vi "run.vi"(8 "error in (no error)":errorcluster, 10 "Path":path, 11 "ConsoleViewer in":refnum<class "ConsoleViewer.lvclass">) -> (0 "error out":errorcluster, 3 "ConsoleViewer out":refnum<class "ConsoleViewer.lvclass">)   [LabVIEW 2009, in "Views.lvlib" / "ConsoleViewer.lvclass"]
uses:
  ConsoleViewer.lvclass
  Tools/CommandProcessor/CommandProcessor.lvclass
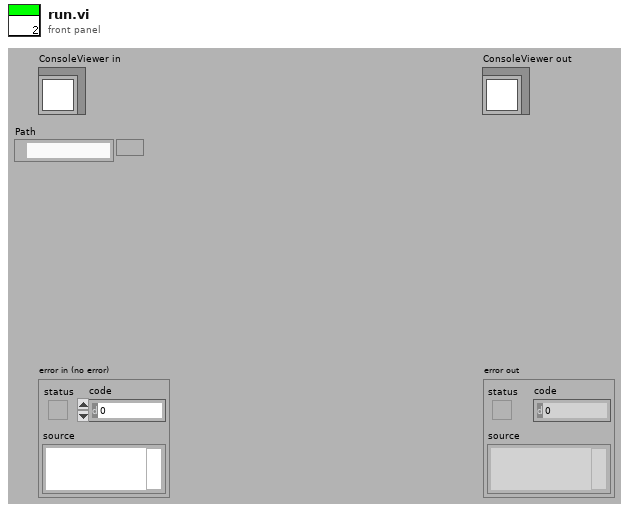
[diagram p1: front panel]
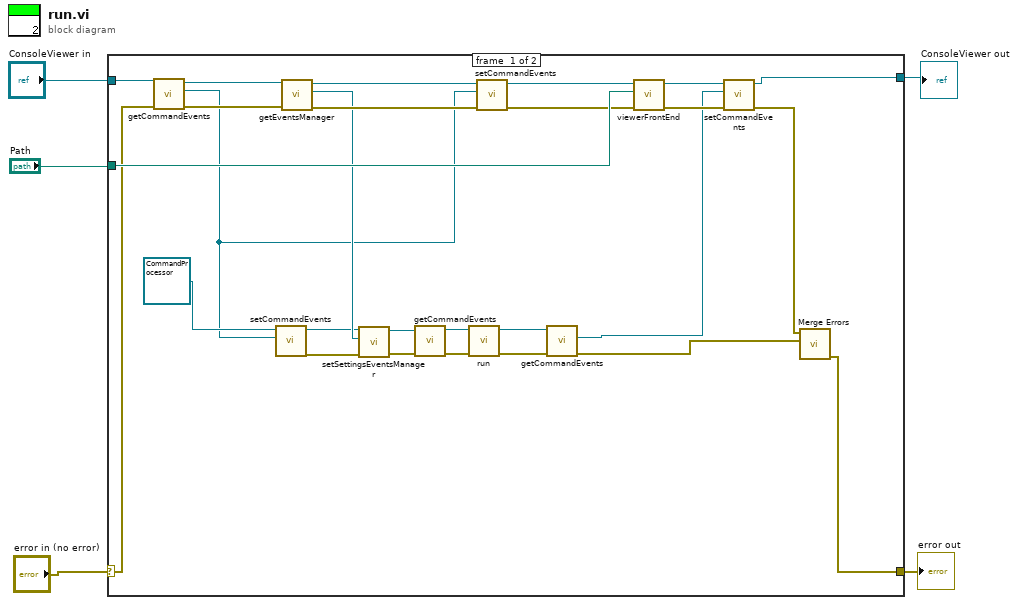
[diagram p0: block diagram]
diagram:
  n1 = case shown="No Error" "error in (no error)" {
    selector: "error in (no error)" -> [w17 w33]
    tunnel: "ConsoleViewer in" -> [w18 w34]
    tunnel: [w9 w34] -> w4
    tunnel: "Path" -> [w32 _]
    tunnel: [w31 w33] -> w1
    frame #0 {
      n2 = call-dynamic "getCommandEvents.vi"("error in (no error)"=w17, "ConsoleViewer.lvclass in"=w18) -> ("error out"=w16:errorcluster, "Tools.lvlib:Interpreters.lvlib:CommandEvents.lvclass"=w6:refnum<class "CommandEvents.lvclass">, "ConsoleViewer.lvclass out"=w15:refnum<class "ConsoleViewer.lvclass">)  [unwired: 7 in]
      n3 = call-dynamic "setCommandEvents.vi"("Tools.lvlib:Interpreters.lvlib:CommandEvents.lvclass"=w6, "CommandProcessor.lvclass in"=refnum<class "CommandProcessor.lvclass"> refnum ("Tools.lvlib:Interpreters.lvlib:CommandProcessor.lvclass")) -> ("error out"=w20:errorcluster, "CommandProcessor.lvclass out"=w21:refnum<class "CommandProcessor.lvclass">)  [unwired: 8 in]
      n4 = call-dynamic "getEventsManager.vi"("error in (no error)"=w16, "SettingsViewer.lvclass in"=w15) -> ("error out"=w26:errorcluster, "Tools.lvlib:Settings.lvlib:SettingsEventsManager.lvclass"=w22:refnum<class "SettingsEventsManager.lvclass">, "SettingsViewer.lvclass out"=w25:refnum<class "ConsoleViewer.lvclass">)  [unwired: 7 in]
      n5 = call-dynamic "setSettingsEventsManager.vi"("error in (no error)"=w20, "Tools.lvlib:Settings.lvlib:SettingsEventsManager.lvclass"=w22, "CommandProcessor.lvclass in"=w21) -> ("error out"=w23:errorcluster, "CommandProcessor.lvclass out"=w24:refnum<class "CommandProcessor.lvclass">)  [unwired: 7 in]
      n6 = call-dynamic "getCommandEvents.vi"("error in (no error)"=w23, "CommandProcessor.lvclass in"=w24) -> ("error out"=w28:errorcluster, "CommandProcessor.lvclass out"=w29:refnum<class "CommandProcessor.lvclass">)  [unwired: 7 in, 1 out]
      n7 = call-dynamic "run.vi"("error in (no error)"=w28, "CommandProcessor in"=w29) -> ("error out"=w8:errorcluster, "CommandProcessor out"=w27:refnum<class "CommandProcessor.lvclass">)  [unwired: 8 in]
      n8 = call-dynamic "setCommandEvents.vi"("error in (no error)"=w26, "Tools.lvlib:Interpreters.lvlib:CommandEvents.lvclass"=w6, "ConsoleViewer.lvclass in"=w25) -> ("error out"=w7:errorcluster, "ConsoleViewer.lvclass out"=w30:refnum<class "ConsoleViewer.lvclass">)  [unwired: 7 in]
      n9 = call-dynamic "getCommandEvents.vi"("error in (no error)"=w8, "CommandProcessor.lvclass in"=w27) -> ("error out"=w14:errorcluster, "Tools.lvlib:Interpreters.lvlib:CommandEvents.lvclass"=w10:refnum<class "CommandEvents.lvclass">)  [unwired: 7 in, 1 out]
      n10 = call-dynamic "viewerFrontEnd.vi"("error in (no error)"=w7, "defaultPath"=w32, "ConsoleViewer in"=w30) -> ("error out"=w12:errorcluster, "ConsoleViewer out"=w13:refnum<class "ConsoleViewer.lvclass">)  [unwired: 7 in]
      n11 = call-dynamic "setCommandEvents.vi"("error in (no error)"=w12, "Tools.lvlib:Interpreters.lvlib:CommandEvents.lvclass"=w10, "ConsoleViewer.lvclass in"=w13) -> ("error out"=w11:errorcluster, "ConsoleViewer.lvclass out"=w9:refnum<class "ConsoleViewer.lvclass">)  [unwired: 7 in]
      n12 = call <vilib>:"Merge Errors.vi"("error in 2 (no error)"=w14, "error in 1 (no error)"=w11) -> ("error out"=w31:errorcluster)  [unwired: 5 in]
    }
    frame #1 {
    }
  }
  "error out" <- w1
  "ConsoleViewer out" <- w4
